vi "Fast Get Item Data FuncGlobal.vi"(5 "Action":enum16{"Open or Add", "Close Ref"}(ring), 8 "error in (no error)":errorcluster, 11 "Item Ref in":T2 format="%.0x") -> (0 "error out":errorcluster, 2 "Item Info":T1, 3 "Item Ref out":T2 format="%.0x", 4 "Found":bool)   [LabVIEW 2011]
doc: "Returns information about the specified item, including the name of the item, the GUID, and whether the item is a channel."
uses:
  <vilib>/NI Veristand/Custom Device API/Custom Device Item Ref.ctl
  <vilib>/NI Veristand/Custom Device API/Custom Device API.lvlib
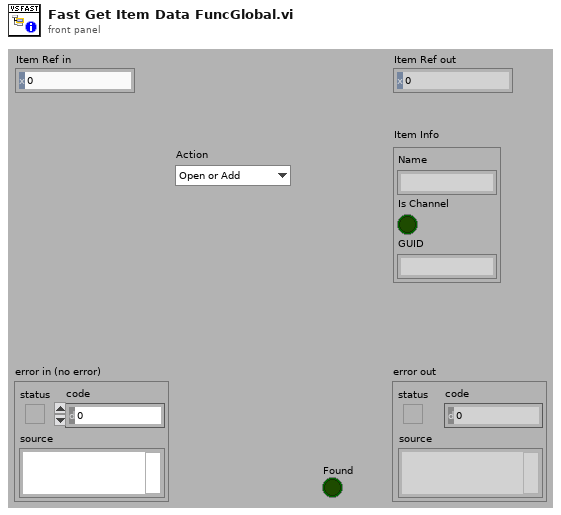
[diagram p1: front panel]
types:
  T1 = cluster{"Name":string, "Is Channel":bool, "GUID":string}
  T2 = typedef "Custom Device API.lvlib/Custom Device Item Ref.ctl" = u64
  T3 = typedef "Custom Device API.lvlib/Custom Device Item Info.ctl" = cluster{"Name":string, "Is Channel":bool, "GUID":string}
  T4 = typedef "Custom Device API.lvlib/Custom Device Item Info.ctl" = cluster{"Name":string, "Is Channel":bool, "GUID":string, "Is Waveform":bool}
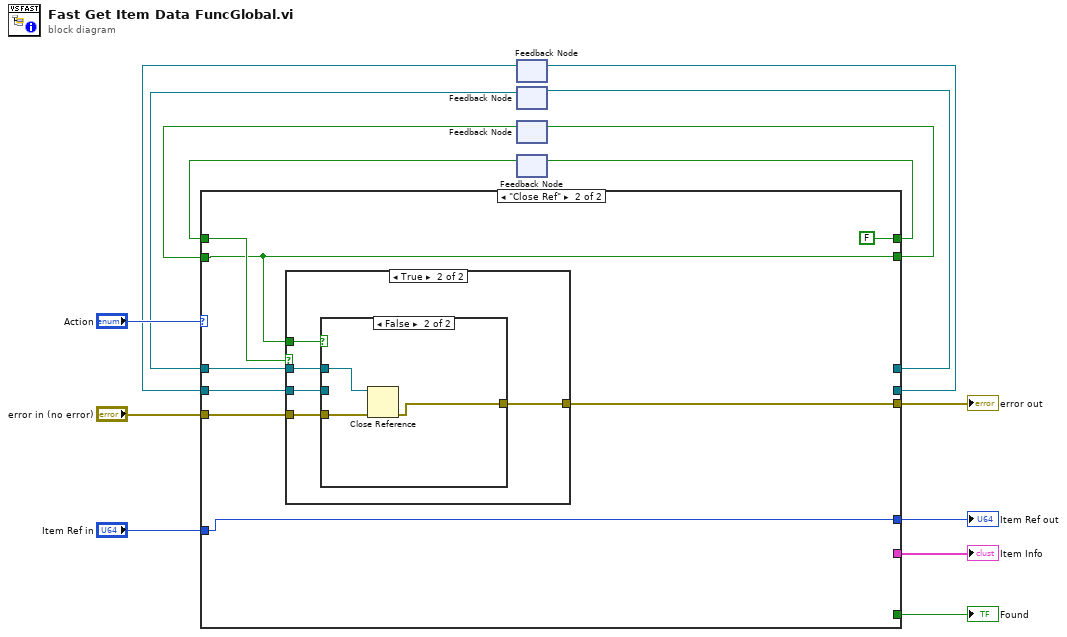
[diagram p0: block diagram]
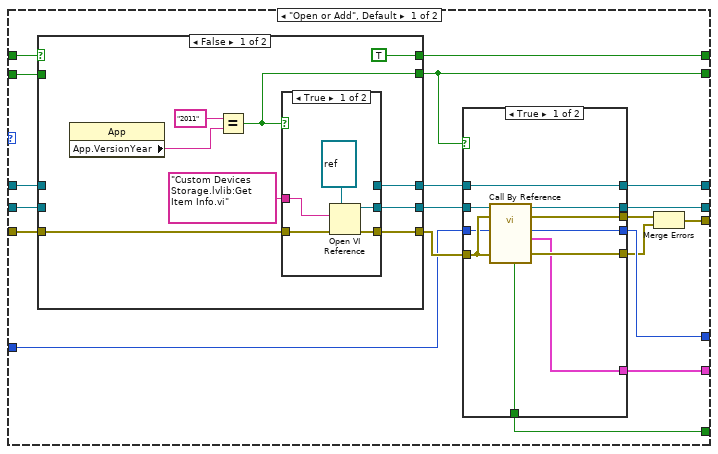
[diagram p2: hidden frame]
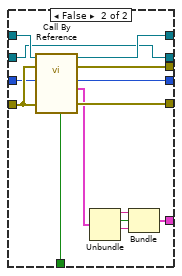
[diagram p3: hidden frame]
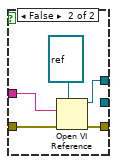
[diagram p4: hidden frame]
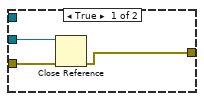
[diagram p7: hidden frame]
diagram:
  n1 = feedback #1() -> (w12:refnum<vi>)  [unwired: 1 in]
  n2 = feedback #2() -> (w1:refnum<vi>)  [unwired: 1 in]
  n3 = feedback #3() -> (w2:bool)  [unwired: 1 in]
  n4 = feedback #4() -> (w10:bool)  [unwired: 1 in]
  n5 = case shown="\"Close Ref\"" "Action" {
    tunnel: "error in (no error)" -> [w34 w90]
    tunnel: [w22 w87] -> w6
    tunnel: [w31 _] -> w13
    tunnel: w12 -> [w30 w89]
    tunnel: [w29 FALSE] -> w11
    tunnel: w10 -> [w28 w88]
    tunnel: "Item Ref in" -> [w27 w85]
    tunnel: [w26 w85] -> w8
    tunnel: [w25 _] -> w7
    tunnel: [w21 w84] -> w3
    tunnel: [w19 _] -> w4
    tunnel: [w18 _] -> w5
    tunnel: w2 -> [w17 w84]
    tunnel: w1 -> [w16 w83]
    frame "Open or Add", Default {
      n6 = case shown="False" w28 {
        selector: w28 -> [_ w80]
        tunnel: w34 -> [w67 w81]
        tunnel: [w66 w81] -> w33
        tunnel: [w65 w82] -> w32
        tunnel: w30 -> [_ w82]
        tunnel: [TRUE w80] -> w29
        tunnel: [w62 w78] -> w20
        tunnel: [w59 w79] -> w21
        tunnel: w17 -> [_ w79]
        tunnel: w16 -> [_ w78]
        frame False {
          n7 = property class="App"() -> ("App.VersionYear"=w61:string)  [unwired: 2 in, 2 out]
          n8 = Equal?(x="2011", y=w61) -> (x = y?=w59:bool)
          n9 = case shown="True" w59 {
            tunnel: w67 -> [w71 w76]
            tunnel: [w70 w75] -> w66
            tunnel: [w69 _] -> w65
            tunnel: "Custom Devices Storage.lvlib:Get Item Info.vi" -> [w68 w74]
            tunnel: [_ w73] -> w62
            frame True {
              n10 = Open VI Reference(type specifier VI Refnum (for type only)=refnum<vi> refnum, vi path=w68, error in (no error)=w71) -> (vi reference=w69:refnum<vi>, error out=w70:errorcluster)  [unwired: 3 out]
            }
            frame False {
              n11 = Open VI Reference(type specifier VI Refnum (for type only)=refnum<vi> refnum, vi path=w74, error in (no error)=w76) -> (vi reference=w73:refnum<vi>, error out=w75:errorcluster)  [unwired: 3 out]
            }
          }
        }
        frame True {
        }
      }
      n12 = case shown="True" w21 {
        tunnel: w33 -> [w44 w58]
        tunnel: w32 -> [w43 w45]
        tunnel: [w42 w45] -> w31
        tunnel: w27 -> [w41 w57]
        tunnel: [w40 w56] -> w26
        tunnel: [w39 w55] -> w25
        tunnel: [w38 w54] -> w24
        tunnel: [w37 w53] -> w23
        tunnel: w20 -> [w35 w52]
        tunnel: [w35 w51] -> w19
        tunnel: [w36 w46] -> w18
        frame True {
          n13 = call-by-ref "?"(reference=w43, error in=w44, 8:"error in (no error)"=w44, "Item Ref in"=w41) -> (reference out=w42:refnum<vi>, error out=w37:errorcluster, 0:"error out"=w38:errorcluster, "Item Info"=w36:T3, "Item Ref out"=w40:T2, "Found"=w39:bool)  [unwired: 6 in]
        }
        frame False {
          n14 = call-by-ref "?"(reference=w52, error in=w58, 8:"error in (no error)"=w58, "Item Ref in"=w57) -> (reference out=w51:refnum<vi>, error out=w53:errorcluster, 0:"error out"=w54:errorcluster, "Item Info"=w50:T4, "Item Ref out"=w56:T2, "Found"=w55:bool)  [unwired: 6 in]
          n15 = Unbundle(w50) -> ("Name"=w49:string, "Is Channel"=w48:bool, "GUID"=w47:string)  [unwired: 1 out]
          n16 = Bundle("Name"=w49, "Is Channel"=w48, "GUID"=w47) -> (w46:T1)  [unwired: 1 in]
        }
      }
      n17 = Merge Errors(w23, w24) -> (w22:errorcluster)
    }
    frame "Close Ref" {
      n18 = case shown="True" w88 {
        tunnel: w90 -> [w91 w96]
        tunnel: w89 -> [_ w95]
        tunnel: [w91 w94] -> w87
        tunnel: w84 -> [_ w93]
        tunnel: w83 -> [_ w92]
        frame False {
        }
        frame True {
          n19 = case shown="False" w93 {
            tunnel: w96 -> [w99 w102]
            tunnel: w95 -> [w98 _]
            tunnel: [w97 w101] -> w94
            tunnel: w92 -> [_ w100]
            frame True {
              n20 = Close Reference(reference=w98, error in (no error)=w99) -> (error out=w97:errorcluster)
            }
            frame False {
              n21 = Close Reference(reference=w100, error in (no error)=w102) -> (error out=w101:errorcluster)
            }
          }
        }
      }
    }
  }
  "error out" <- w6
  "Item Ref out" <- w8
  "Found" <- w7
  "Item Info" <- w5
  n22 = feedback-in #1(w13) -> ()
  n23 = feedback-in #2(w4) -> ()
  n24 = feedback-in #3(w3) -> ()
  n25 = feedback-in #4(w11) -> ()
